vi "DROPBEAR_Model_Updating_Pack_Data.vi"(9 "Timing stats":T3, 10 "Signal Quality":T2, 11 "Setup Parameters and Controls":T1={"Modeling Parameters input controls"={"beam_length"=0.0, "youngs_modulus"=0.0, "torsion_spring"=0.0, "beam_height"=0.0, "beam_width"=0.0, "beam_density"=0.0, "number_of_FEA_nodes"=0, "accelerometer_mass"=0.0}, "Mockbear input controls"={"Dataset"="", "Resample Method"=enum."Recorded"}, "Simulation Parameters input controls"={"Eigensolver "=enum."LEMP", "Models Forcasted"=0, "Max Roller Velocity"=0.0, "Max Roller Position Percent"=0.43, "Min Roller Position Percent"=0.155}, "Program Controls"={"Frequency KF"=TRUE, "Pinned State KF"=TRUE, "FFT Bounding"=TRUE, "Filter Constants Frequency"={"Measurement Variance"=0.0, "State Variance"=0.0, "Threshold"=0.0}, "Filter Constants Position"={"Measurement Variance"=0.0, "State Variance"=0.0, "Threshold"=0.0}, "Moving Window Size"=0, "Time Series buffer"=0.0, "Record Time Series Data"=FALSE, "Record Moving Window Data"=FALSE, "Record Online Error Metrics "=FALSE, "Record Statistics"=FALSE}}) -> (3 "String":string)   [LabVIEW 2021, in "DROPBEAR_Model_Updating.lvclass"]
uses:
  DROPBEAR_Model_Updating.lvclass
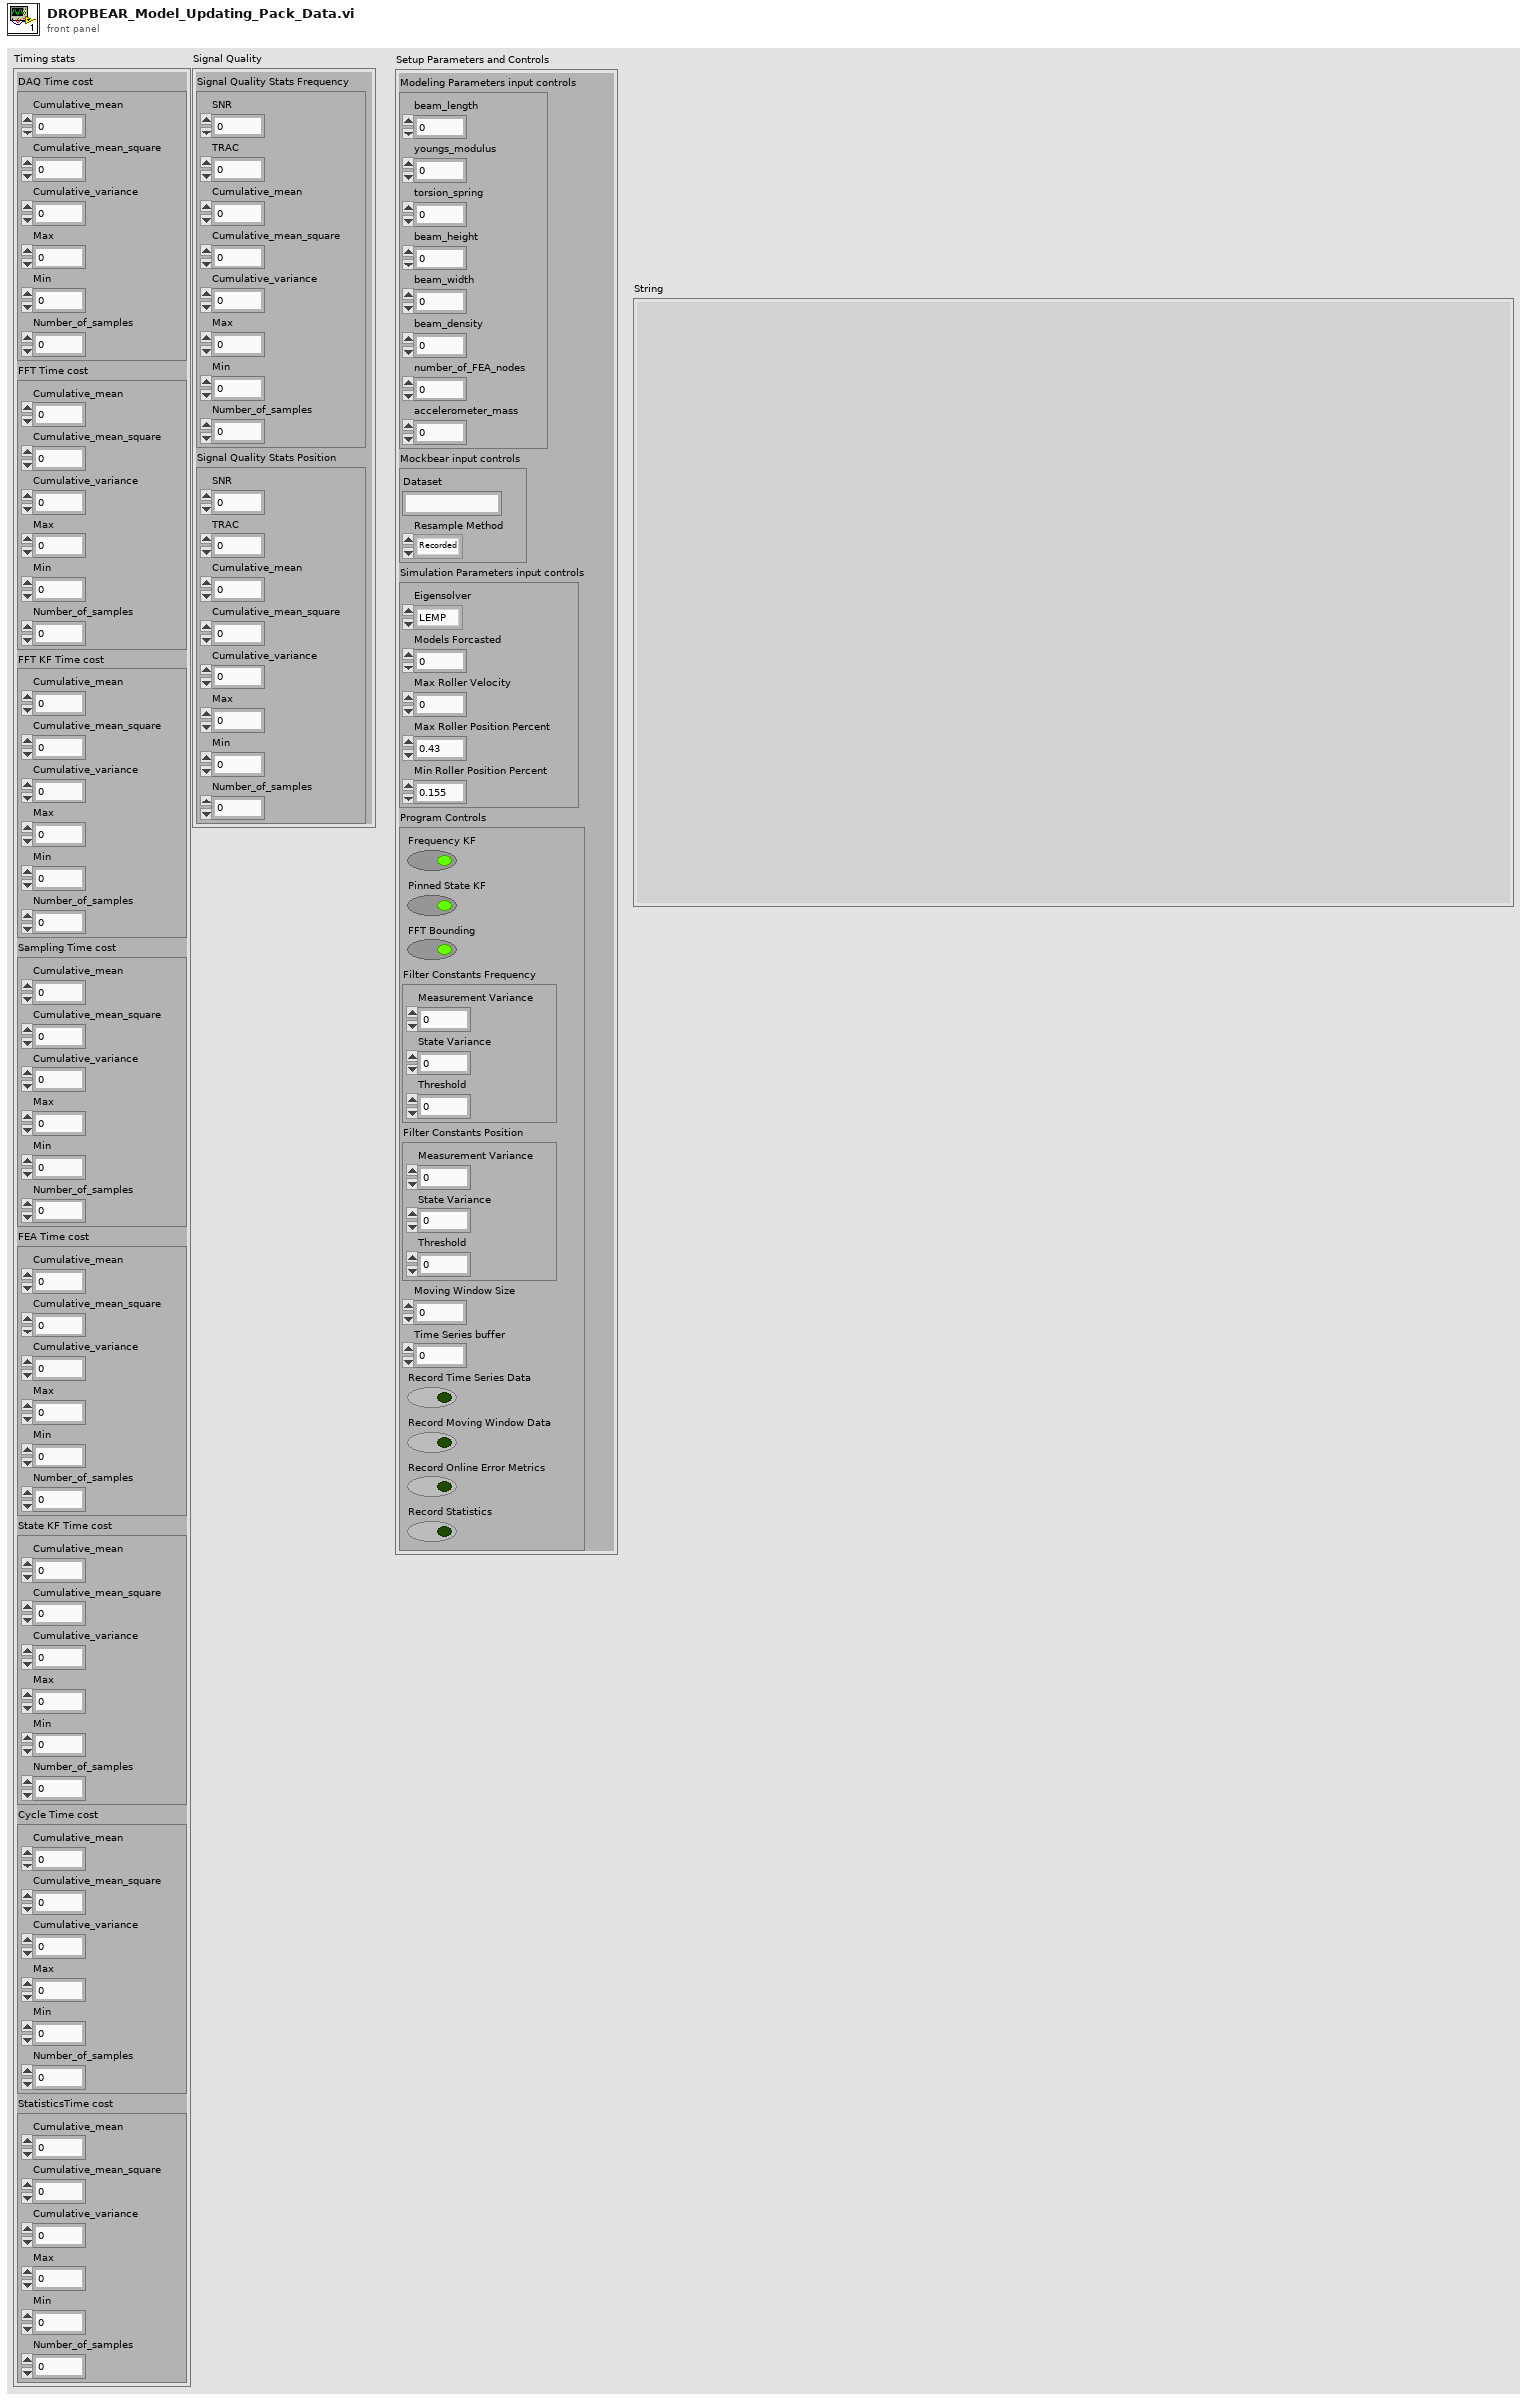
[diagram p1: front panel]
types:
  T1 = cluster{"Modeling Parameters input controls":cluster{"beam_length":dbl, "youngs_modulus":dbl, "torsion_spring":dbl, "beam_height":dbl, "beam_width":dbl, "beam_density":dbl, "number_of_FEA_nodes":i32, "accelerometer_mass":dbl}, "Mockbear input controls":cluster{"Dataset":string, "Resample Method":enum16{"Recorded", "Auto Resample", "Custom Resample"}}, "Simulation Parameters input controls":cluster{"Eigensolver ":enum16{"LabVIEW Cholesky", "LabVIEW General", "LabVIEW Inverse", "LEMP"}, "Models Forcasted":i32, "Max Roller Velocity":dbl, "Max Roller Position Percent":dbl, "Min Roller Position Percent":dbl}, "Program Controls":cluster{"Frequency KF":bool, "Pinned State KF":bool, "FFT Bounding":bool, "Filter Constants Frequency":cluster{"Measurement Variance":dbl, "State Variance":dbl, "Threshold":dbl}, "Filter Constants Position":cluster{"Measurement Variance":dbl, "State Variance":dbl, "Threshold":dbl}, "Moving Window Size":i32, "Time Series buffer":dbl, "Record Time Series Data":bool, "Record Moving Window Data":bool, "Record Online Error Metrics ":bool, "Record Statistics":bool}}
  T2 = cluster{"Signal Quality Stats Frequency":cluster{"SNR":dbl, "TRAC":dbl, "Cumulative_mean":dbl, "Cumulative_mean_square ":dbl, "Cumulative_variance":dbl, "Max":dbl, "Min":dbl, "Number_of_samples":i32}, "Signal Quality Stats Position":cluster{"SNR":dbl, "TRAC":dbl, "Cumulative_mean":dbl, "Cumulative_mean_square ":dbl, "Cumulative_variance":dbl, "Max":dbl, "Min":dbl, "Number_of_samples":i32}}
  T3 = cluster{"DAQ Time cost":cluster{"Cumulative_mean":dbl, "Cumulative_mean_square ":dbl, "Cumulative_variance":dbl, "Max":dbl, "Min":dbl, "Number_of_samples":i32}, "FFT Time cost":cluster{"Cumulative_mean":dbl, "Cumulative_mean_square ":dbl, "Cumulative_variance":dbl, "Max":dbl, "Min":dbl, "Number_of_samples":i32}, "FFT KF Time cost":cluster{"Cumulative_mean":dbl, "Cumulative_mean_square ":dbl, "Cumulative_variance":dbl, "Max":dbl, "Min":dbl, "Number_of_samples":i32}, "Sampling Time cost":cluster{"Cumulative_mean":dbl, "Cumulative_mean_square ":dbl, "Cumulative_variance":dbl, "Max":dbl, "Min":dbl, "Number_of_samples":i32}, "FEA Time cost":cluster{"Cumulative_mean":dbl, "Cumulative_mean_square ":dbl, "Cumulative_variance":dbl, "Max":dbl, "Min":dbl, "Number_of_samples":i32}, "State KF Time cost":cluster{"Cumulative_mean":dbl, "Cumulative_mean_square ":dbl, "Cumulative_variance":dbl, "Max":dbl, "Min":dbl, "Number_of_samples":i32}, "Cycle Time cost":cluster{"Cumulative_mean":dbl, "Cumulative_mean_square ":dbl, "Cumulative_variance":dbl, "Max":dbl, "Min":dbl, "Number_of_samples":i32}, "StatisticsTime cost":cluster{"Cumulative_mean":dbl, "Cumulative_mean_square ":dbl, "Cumulative_variance":dbl, "Max":dbl, "Min":dbl, "Number_of_samples":i32}}
  T4 = enum16{"Recorded", "Auto Resample", "Custom Resample"}
  T5 = enum16{"LabVIEW Cholesky", "LabVIEW General", "LabVIEW Inverse", "LEMP"}
  T6 = cluster{"Cumulative_mean":dbl, "Cumulative_mean_square ":dbl, "Cumulative_variance":dbl, "Max":dbl, "Min":dbl, "Number_of_samples":i32}
  T7 = cluster{"SNR":dbl, "TRAC":dbl, "Cumulative_mean":dbl, "Cumulative_mean_square ":dbl, "Cumulative_variance":dbl, "Max":dbl, "Min":dbl, "Number_of_samples":i32}
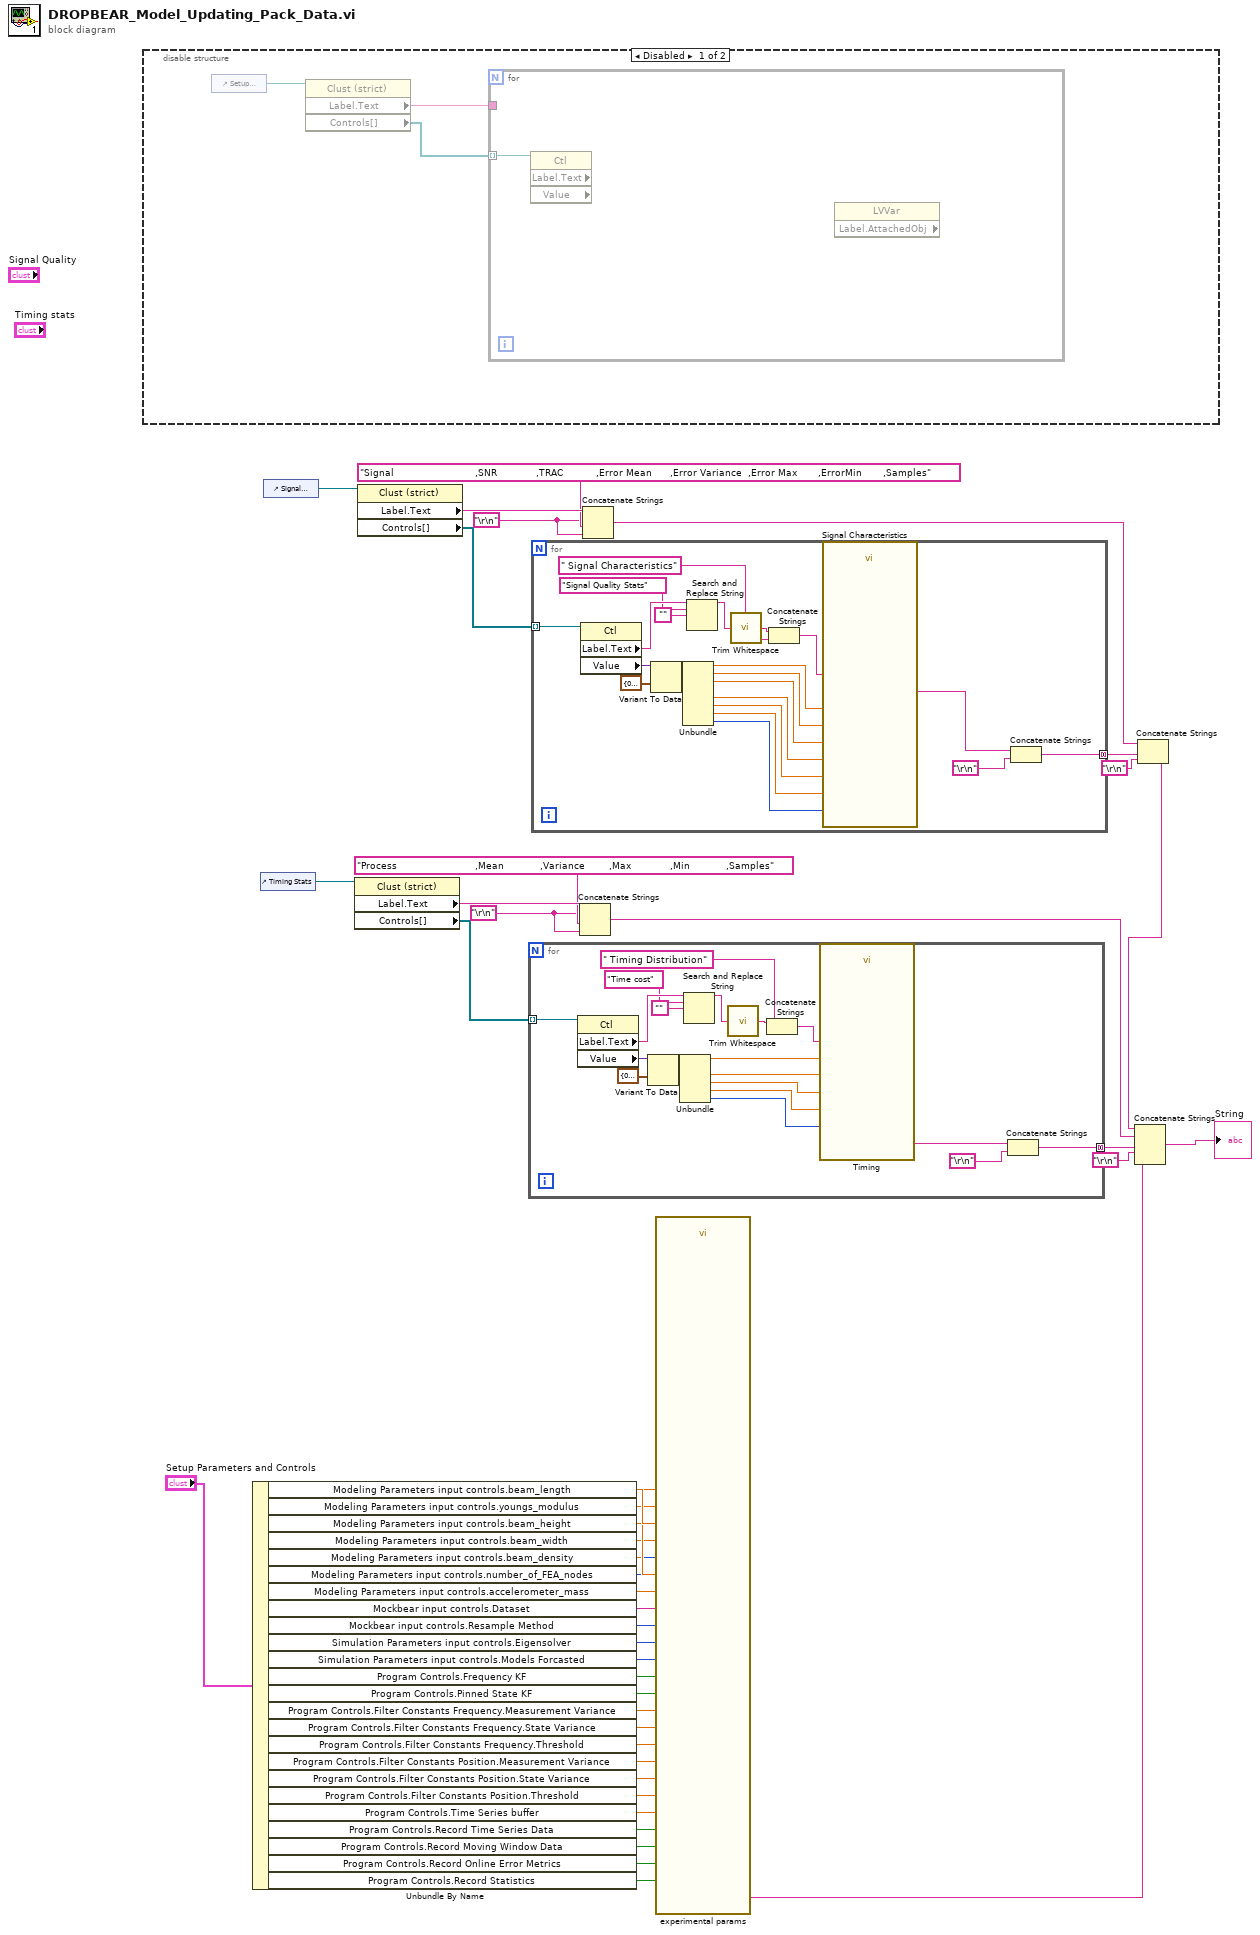
[diagram p0: block diagram]
diagram:
  w32 = "\r\n"
  w40 = "\r\n"
  n1 = disable-structure shown="Disabled" {
    frame Disabled {
      n2 = control-ref of="Setup Parameters and Controls"() -> (w47:refnum<vi>)
      n3 = property class="Clust (strict)"(reference=w47) -> ("Label.Text"=w45:string, "Controls[]"=w46:refnum<vi>[])  [unwired: 1 in, 2 out]
      n4 = for {
        tunnel: w46 -> [w51] mode=indexing
        tunnel: w45 -> [_]
        n5 = property class="Ctl"(reference=w51) -> ("Label.Text"=w50:string, "Value"=w49:variant)  [unwired: 1 in, 2 out]
        n6 = property class="LVVar" props=["Label", "AttachedObj"]() -> (reference=w48:refnum<vi>)  [unwired: 1 in, 3 out]
      }
    }
    frame Enabled {
    }
  }
  n7 = Unbundle By Name("Setup Parameters and Controls") -> ("Modeling Parameters input controls.beam_length"=w26:dbl, "Modeling Parameters input controls.youngs_modulus"=w25:dbl, "Modeling Parameters input controls.beam_height"=w24:dbl, "Modeling Parameters input controls.beam_width"=w23:dbl, "Modeling Parameters input controls.beam_density"=w22:dbl, "Modeling Parameters input controls.number_of_FEA_nodes"=w21:i32, "Modeling Parameters input controls.accelerometer_mass"=w20:dbl, "Mockbear input controls.Dataset"=w19:string, "Mockbear input controls.Resample Method"=w18:T4, "Simulation Parameters input controls.Eigensolver"=w17:T5, "Simulation Parameters input controls.Models Forcasted"=w16:i32, "Program Controls.Frequency KF"=w15:bool, "Program Controls.Pinned State KF"=w3:bool, "Program Controls.Filter Constants Frequency.Measurement Variance"=w4:dbl, "Program Controls.Filter Constants Frequency.State Variance"=w5:dbl, "Program Controls.Filter Constants Frequency.Threshold"=w6:dbl, "Program Controls.Filter Constants Position.Measurement Variance"=w7:dbl, "Program Controls.Filter Constants Position.State Variance"=w8:dbl, "Program Controls.Filter Constants Position.Threshold"=w9:dbl, "Program Controls.Time Series buffer"=w10:dbl, "Program Controls.Record Time Series Data"=w11:bool, "Program Controls.Record Moving Window Data"=w12:bool, "Program Controls.Record Online Error Metrics"=w13:bool, "Program Controls.Record Statistics"=w14:bool)
  n8 = control-ref of="Timing Stats"() -> (w44:refnum<vi>)
  n9 = control-ref of="Signal Quality"() -> (w36:refnum<vi>)
  n10 = property class="Clust (strict)"(reference=w44) -> ("Label.Text"=w42:string, "Controls[]"=w43:refnum<vi>[])  [unwired: 1 in, 2 out]
  n11 = property class="Clust (strict)"(reference=w36) -> ("Label.Text"=w34:string, "Controls[]"=w35:refnum<vi>[])  [unwired: 1 in, 2 out]
  n12 = for {
    tunnel: w43 -> [w70] mode=indexing
    tunnel: [w55] -> w39 mode=concatenating
    n13 = property class="Ctl"(reference=w70) -> ("Label.Text"=w59:string, "Value"=w67:variant)  [unwired: 1 in, 2 out]
    n14 = Variant To Data(type=T6 {"Cumulative_mean"=0.0, "Cumulative_mean_square "=0.0, "Cumulative_variance"=0.0, "Max"=0.0, "Min"=0.0, "Number_of_samples"=0} ("StatisticsTime cost"), Variant=w67) -> (data=w68:T6)  [unwired: 1 in, 1 out]
    n15 = Unbundle(w68) -> ("Cumulative_mean"=w66:dbl, "Cumulative_variance"=w65:dbl, "Max"=w64:dbl, "Min"=w63:dbl, "Number_of_samples"=w62:i32)  [unwired: 1 out]
    n16 = Search and Replace String(input string=w59, search string="Time cost", replace string="") -> (result string=w56:string)  [unwired: 5 in, 3 out]
    n17 = call <vilib>:"Trim Whitespace.vi"("string"=w56) -> ("trimmed string"=w54:string)  [unwired: 1 in]
    n18 = Concatenate Strings(w54, " Timing Distribution" ("string")) -> (w53:string)
    n19 = call "Timing"("Max"=w64, "Num_Samples"=w62, "Statistic"=w53, "Mean"=w66, "Variance"=w65, "Min"=w63) -> ("Result"=w61:string)  [unwired: 8 in, 1 out]
    n20 = Concatenate Strings(w61, "\r\n") -> (w55:string)
  }
  n21 = for {
    tunnel: w35 -> [w91] mode=indexing
    tunnel: [w82] -> w31 mode=concatenating
    n22 = property class="Ctl"(reference=w91) -> ("Label.Text"=w86:string, "Value"=w89:variant)  [unwired: 1 in, 2 out]
    n23 = Variant To Data(type=T7 {"SNR"=0.0, "TRAC"=0.0, "Cumulative_mean"=0.0, "Cumulative_mean_square "=0.0, "Cumulative_variance"=0.0, "Max"=0.0, "Min"=0.0, "Number_of_samples"=0} ("Signal Quality Stats Frequency"), Variant=w89) -> (data=w90:T7)  [unwired: 1 in, 1 out]
    n24 = Unbundle(w90) -> ("SNR"=w80:dbl, "TRAC"=w79:dbl, "Cumulative_mean"=w78:dbl, "Cumulative_variance"=w77:dbl, "Max"=w76:dbl, "Min"=w75:dbl, "Number_of_samples"=w74:i32)  [unwired: 1 out]
    n25 = Search and Replace String(input string=w86, search string="Signal Quality Stats", replace string="") -> (result string=w83:string)  [unwired: 5 in, 3 out]
    n26 = call <vilib>:"Trim Whitespace.vi"("string"=w83) -> ("trimmed string"=w73:string)  [unwired: 1 in]
    n27 = Concatenate Strings(w73, " Signal Characteristics") -> (w72:string)
    n28 = call "Signal Characteristics"("Mean"=w78, "Max"=w76, "Num_Samples"=w74, "Statistic"=w72, "SNR"=w80, "TRAC"=w79, "Variance"=w77, "Min"=w75) -> ("Result"=w88:string)  [unwired: 6 in, 1 out]
    n29 = Concatenate Strings(w88, "\r\n") -> (w82:string)
  }
  n30 = Concatenate Strings(w42, w40, "Process                          ,Mean            ,Variance        ,Max             ,Min            ,Samples", w40) -> (w37:string)
  n31 = Concatenate Strings(w34, w32, "Signal                           ,SNR             ,TRAC           ,Error Mean      ,Error Variance  ,Error Max       ,ErrorMin       ,Samples", w32) -> (w30:string)
  n32 = call "experimental params"("beamlength"=w26, "youngsmodulus"=w25, "beamheight"=w24, "beamwidth"=w23, "beamdensity"=w22, "FEANodes"=w21, "accelmass"=w20, "dataset"=w19, "resamplemethod"=w18, "ES"=w17, "MF"=w16, "FrequencyKF"=w15, "StateKF"=w3, "fmv"=w4, "fsv"=w5, "fthresh"=w6, "smv"=w7, "ssv"=w8, "sthresh"=w9, "buff"=w10, "rtime"=w11, "rmv"=w12, "rom"=w13, "rts"=w14) -> ("Result"=w1:string)  [unwired: 2 in, 1 out]
  n33 = Concatenate Strings(w30, w31, "\r\n") -> (w28:string)
  n34 = Concatenate Strings(w28, w37, w39, "\r\n", w1) -> (→"String":string)
